vi "FP Position.vi"(9 "Module ID":i32, 10 "error in":errorcluster, 11 "VI server in":refnum<vi>) -> ()   [LabVIEW 2021, in "Slave.lvlib"]
uses:
  Slave.lvlib
  <vilib>/Utility/miscctls.llb/LVRectTypeDef.ctl
panel:
  out "WinBounds":T1
  out "Size":cluster{"Height":i16, "Width":i16}
  out "Type":T2(ring)
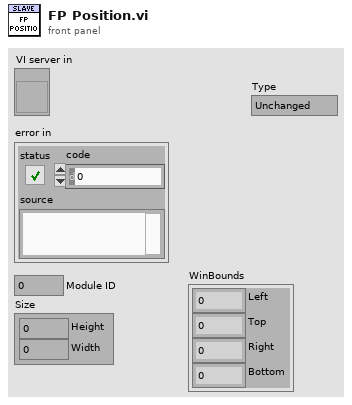
[diagram p1: front panel]
types:
  T1 = typedef "LVRectTypeDef.ctl" = cluster{"Left":i16, "Top":i16, "Right":i16, "Bottom":i16}
  T2 = enum32{"Unchanged", "Centered", "Maximized", "Minimized", "Custom"}
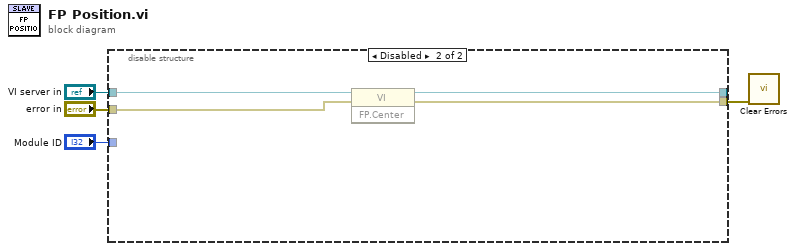
[diagram p0: block diagram]
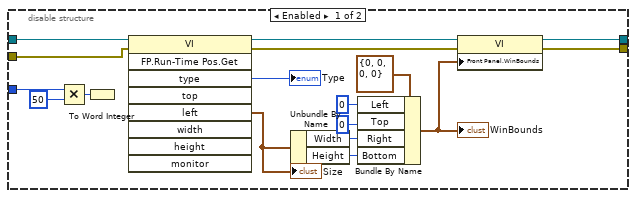
[diagram p2: hidden frame]
diagram:
  n1 = disable-structure shown="Disabled" {
    disable-tunnel: "VI server in" -> [w21 w25]
    disable-tunnel: "Module ID" -> [w20 _]
    disable-tunnel: [w15 w22] -> _
    disable-tunnel: [w5 w23] -> w1
    disable-tunnel: "error in" -> [w14 w24]
    frame Enabled {
      n2 = Multiply(x=w20, y=50) -> (x*y=w18:i32)
      n3 = To Word Integer(number=w18) -> ()  [unwired: 1 out]
      n4 = invoke class="VI" method="FP.Run-Time Pos.Get"(reference=w21, error in=w14) -> (reference out=w17:refnum<vi>, error out=w16:errorcluster, "type"=→"Type":T2, "left"=w8:cluster{"Height":i16, "Width":i16})  [unwired: 7 in, 5 out]
      "Size" <- w8
      n5 = Unbundle By Name(w8) -> ("Width"=w6:i16, "Height"=w7:i16)
      n6 = Bundle By Name(cluster=T1 {"Left"=0, "Top"=0, "Right"=0, "Bottom"=0} ("Front Panel Window:Window Bounds"), "Left"=i16 0, "Top"=i16 0, "Right"=w6, "Bottom"=w7) -> (w11:T1)
      "WinBounds" <- w11
      n7 = property class="VI"(reference=w17, error in=w16, "Front Panel.WinBounds"=w11) -> (reference out=w15:refnum<vi>, error out=w5:errorcluster)
    }
    frame Disabled {
      n8 = invoke class="VI" method="FP.Center"(reference=w25, error in=w24) -> (reference out=w22:refnum<vi>, error out=w23:errorcluster)  [unwired: 1 in, 1 out]
    }
  }
  n9 = call <vilib>:"Clear Errors.vi"("error in (no error)"=w1) -> ()  [unwired: 5 in, 2 out]
